vi "Scope_AM_PID_tester.vi"() -> ()   [LabVIEW 2013]
uses:
  <vilib>/rvi/interface/nirviCloseFPGA/nirviCloseFPGA.xnode
  <vilib>/rvi/interface/nirviOpenFPGA/nirviOpenFPGA.xnode
  Scope5782/Config/FPGAref_5782.ctl
  Scope/controls/Data_calc_mode.ctl
  Utilities/Ticker/Ticker.lvclass
  Scope/controls/ScopeMode.ctl
  <vilib>/rvi/interface/nirviReadWriteControl/nirviReadWriteControl.xnode
  <vilib>/Utility/error.llb/Error Cluster From Error Code.vi
  <vilib>/rvi/interface/Simulation/niFpgaSimulationCallBeginRW.vi
  <vilib>/rvi/errors/niLvFpgaAdjustHostInterfaceError.vi
  NiFpgaLv.dll
  Communication/Driver/TcpServerDriver/TcpServerDriver.lvclass
  Communication/driver_status.ctl
  Communication/response.ctl
  Communication/global_stop.vi
  Communication/Driver/RemoteConnection/RemoteConnection.lvclass
  Communication/Driver/RemoteConnection/RemoteReferences.ctl
  FPGA/fpga_settings.ctl
  <vilib>/rvi/interface/nirviMethod/nirviMethod.xnode
  <vilib>/FPGAPlugInAG/Dynamic/niLvFpga_WriteFifo_Dynamic.vi
  <vilib>/rvi/errors/niLvFpgaMergeErrorWithErrorCode.vi
  <vilib>/rvi/FXPMathLib/FxpInterpret/XNode/nifxpmath_Interpret.xnode
  <vilib>/FPGAPlugInAG/Dynamic/niLvFpga_Close_Dynamic.vi
  FPGA/DataMode.ctl
  Scope5782/Scope/controls/5782_trigger_type.ctl
  FPGA Bitfiles/AM_PID_tester_3_LzNp9O2tiLo.lvbitx
  <vilib>/FPGAPlugInAG/PXIe-7975R/niLvFpga_Open_PXIe-7975R.vi
  <vilib>/rvi/interface/common/dynamic/niFpgaDynamicAddResources.vi
  <vilib>/userdefined/High Color/nirio_resource_hc.ctl
  <vilib>/Analysis/4window.llb/windowTd.ctl
  <vilib>/Analysis/NI_AALPro.lvlib
  Scope/controls/power_spectrum_unit.ctl
  Scope/controls/graph_controls.ctl
  Scope/controls/Graph_references.ctl
  Scope/controls/Channel_select.ctl
  Scope/controls/Data_display_mode.ctl
panel:
  in  "frequency [MHz]":dbl=0.04
  in  "Ch1 deltaF":bool
  in  "c(t)":bool
  in  "Kp":fxp<+/-,32,4>
  in  "Kd/T":fxp<+/-,32,4>
  in  "Ki*T":fxp<+/-,32,4>
  in  "Feedback":bool
  in  "#bins":i32=1 min=1 max=16
  in  "Chart length":i32=200000
  in  "Trigmode":enum32{"Triggered", "Continuous"}(radio)
  in  "Refence for phase":T1
  in  "Graph_refs":T2
  out "Lower chart":dbl[][](graph)
  out "Upper chart":dbl[][](graph)
  out "Lower graph":i16[][](graph)
  in  "Buffer":T4
  in  "Display":T5
  in  "Ch1 Q":bool
  in  "Ch1 I":bool
  in  "Ch0 Q":bool
  in  "Ch0 I":bool
  in  "Ch1":bool
  in  "Ch0":bool
  out "stop 2":bool
  in  "Zoom freq X":bool
  in  "Zoom freq Y":bool
  in  "Zoom time Y":bool
  in  "Zoom time X":bool
  in  "Unit":T6
  in  "Window":T7=1 items=["Rectangle"=0, "Hanning"=1, "Hamming"=2, "Blackman-Harris"=3, "Exact Blackman"=4, "Blackman"=5, "Flat Top"=6, "4 Term B-Harris "=7, "7 Term B-Harris"=8, "Low Sidelobe"=9, "Blackman Nuttall"=11, "Triangle"=30, "Bartlett-Hanning"=31, "Bohman"=32, "Parzen"=33, "Welch"=34, "Kaiser"=60, "Dolph-Chebyshev"=61, "Gaussian"=62]
  in  "Samples per 5782 record":i32
  out "freqdata":cluster{"f0":dbl, "df":dbl, "magnitude":dbl[]}[](graph)
  out "Upper graph":i16[][](graph)
  in  "Rumode":bool
  in  "Singleshot":bool
  out "error IO":errorcluster
  in  "stop":bool
  in  "resource name":T8="RIO0"
  out "Clocking Option Configured?":bool
  out "Configured?":bool
  # "Auto Zoom"
  # "5782"
  # "FFT"
  # "Auto Zoom"
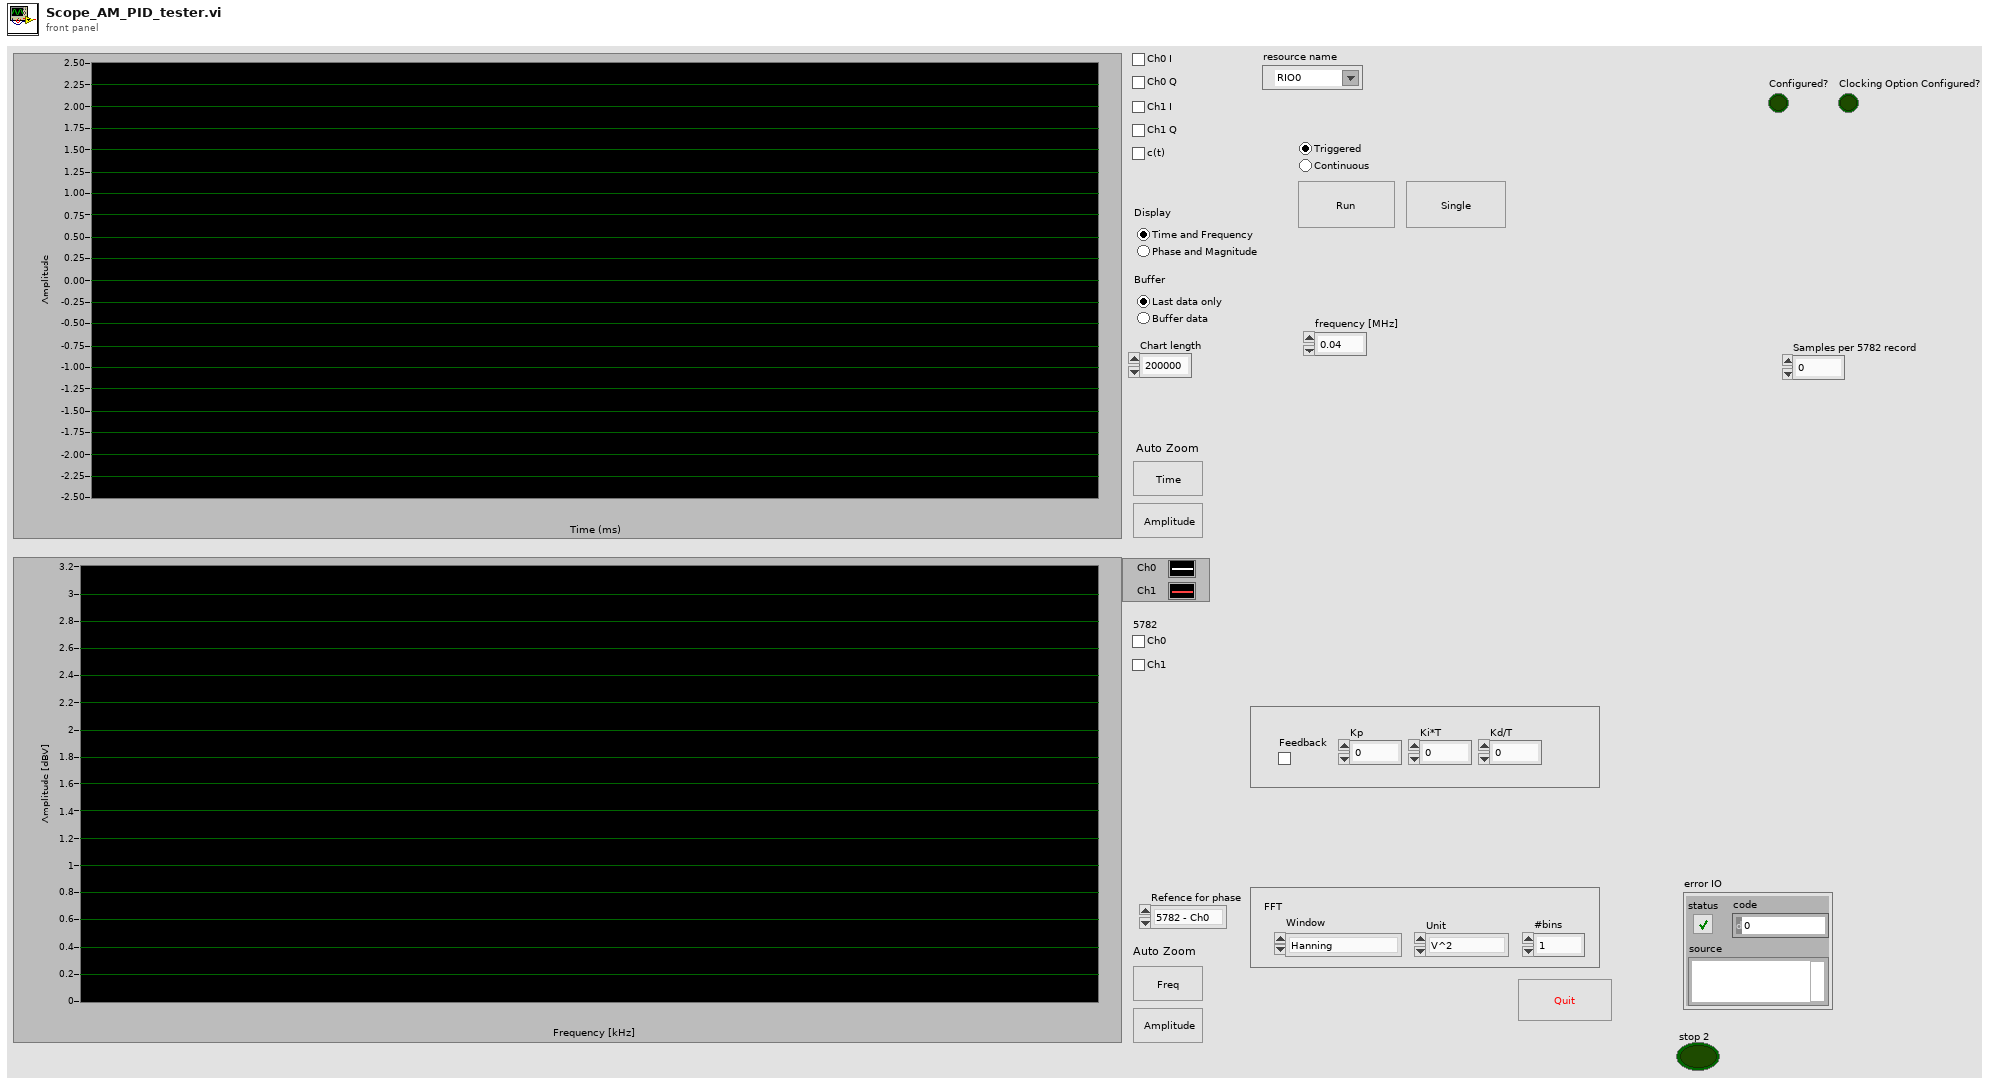
[diagram p1: front panel]
types:
  T1 = typedef "Channel_select.ctl" = enum16{"5782 - Ch0", "5782 - Ch1"}
  T2 = typedef "Graph_references.ctl" = cluster{"upper":T3, "lower":T3, "Freq graph":refnum<vi>}
  T3 = typedef "graph_controls.ctl" = cluster{"Graph":refnum<vi>, "Time btn":refnum<vi>, "Amplitude btn":refnum<vi>, "Chart":refnum<vi>}
  T4 = typedef "Data_display_mode.ctl" = enum32{"Last data only", "Buffer data"}
  T5 = typedef "Data_calc_mode.ctl" = enum32{"Time and Frequency", "Phase and Magnitude"}
  T6 = typedef "power_spectrum_unit.ctl" = enum16{"V^2", "V", "dBV"}
  T7 = typedef "NI_AALPro.lvlib/windowTd.ctl" = u32
  T8 = typedef "nirio_resource_hc.ctl" = tag
  T9 = typedef "5782_trigger_type.ctl" = enum16{"Software", "Trigger input"}
  T10 = typedef "DataMode.ctl" = enum16{"Real IO", "Simulated"}
  T11 = typedef "RemoteConnection.lvclass/RemoteReferences.ctl" = cluster{"a":refnum<vi>, "b":refnum<vi>, "fm":refnum<vi>, "Output delay":refnum<vi>, "Output delay delta":refnum<vi>}
  T12 = typedef "response.ctl" = cluster{"driver status":T13, "Sender":string, "Type":i32, "Variant":variant}
  T13 = typedef "driver_status.ctl" = enum16{"Normal", "Startup", "Connection lost", "Reconnected", "Timeout", "Idle", "Busy"}
  T14 = enum8{"Internal Clock PLL Off", "Internal Clock PLL On (REF IN)", "External Clock (CLK_IN)", "Internal Clock PLL On (IoModSyncClk)"}
  T15 = typedef "message_queue.ctl" = refnum<queue>
  T16 = typedef "FPGAref_config.ctl" = refnum<k20>
  T17 = typedef "FPGAref_5782.ctl" = refnum<k20>
  T18 = typedef "FPGAref_5782_DMA.ctl" = refnum<k20>
  T19 = typedef "scope_params_5782.ctl" = cluster{"scope mode":T20, "ticker":refnum<class "Ticker.lvclass">, "samples per record":i32, "FPGA ref":T17, "data mode":T10, "5782 Trigger":T9, "Chart length":i32, "RemoteConnection":refnum<class "RemoteConnection.lvclass">, "last phase":dbl[]}
  T20 = typedef "ScopeMode.ctl" = enum16{"Stopped", "Single", "Running", "Continuous"}
  T21 = typedef "fpga_settings.ctl" = enum16{"Feedback Enable", "New FIR coeffs", "FIR shift", "Enable filter", "Set Downsample", "Downsample", "CIC Gain", "Record length", "Trigger samples", "Quiet time", "a_am", "b_am", "Use fixed delay", "fixed sin_fi", "fixed cos_fi", "Ki*Tau", "Kp", "Kd_Tau", "Fi_start", "Fi_delta", "DC_offs 0", "DC_offs 1", "DC_offs 2", "DC_offs 3", "Ki*Tau am", "Kp am", "Kd_Tau am", "Feedback AM"}
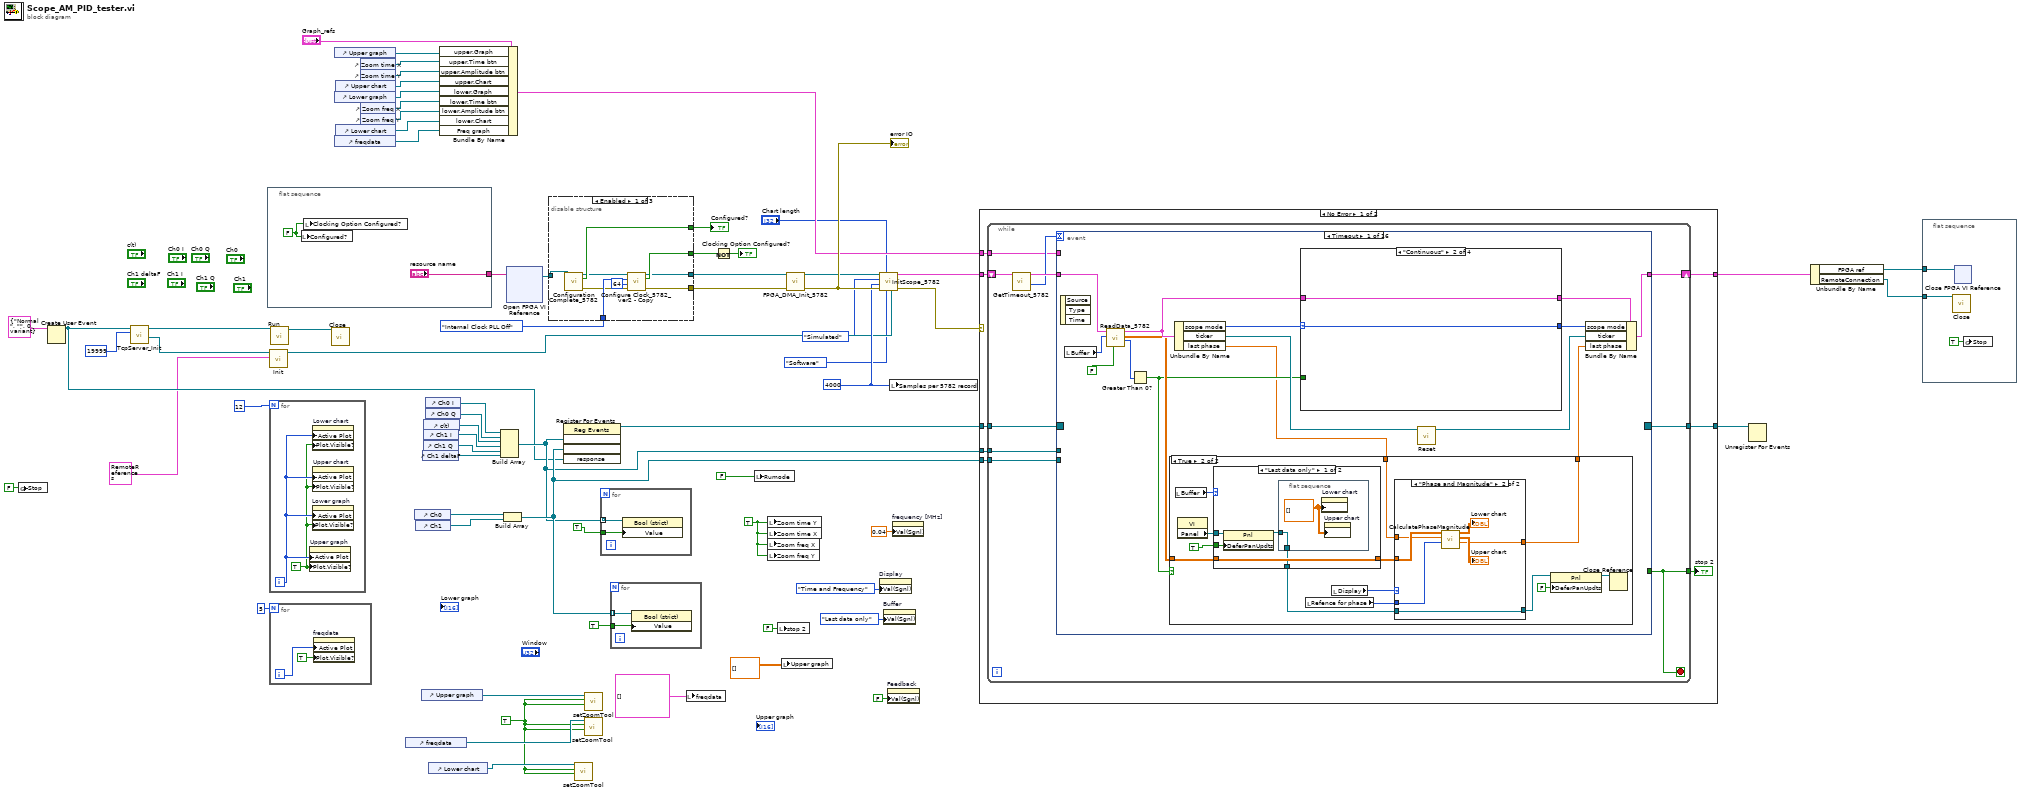
[diagram p0: block diagram]
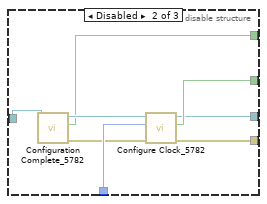
[diagram p2: hidden frame]
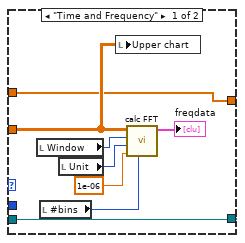
[diagram p6: hidden frame]
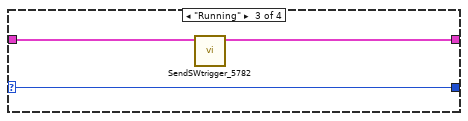
[diagram p8: hidden frame]
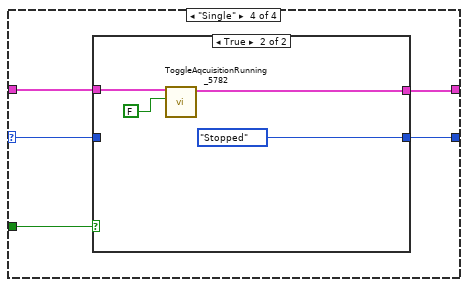
[diagram p9: hidden frame]
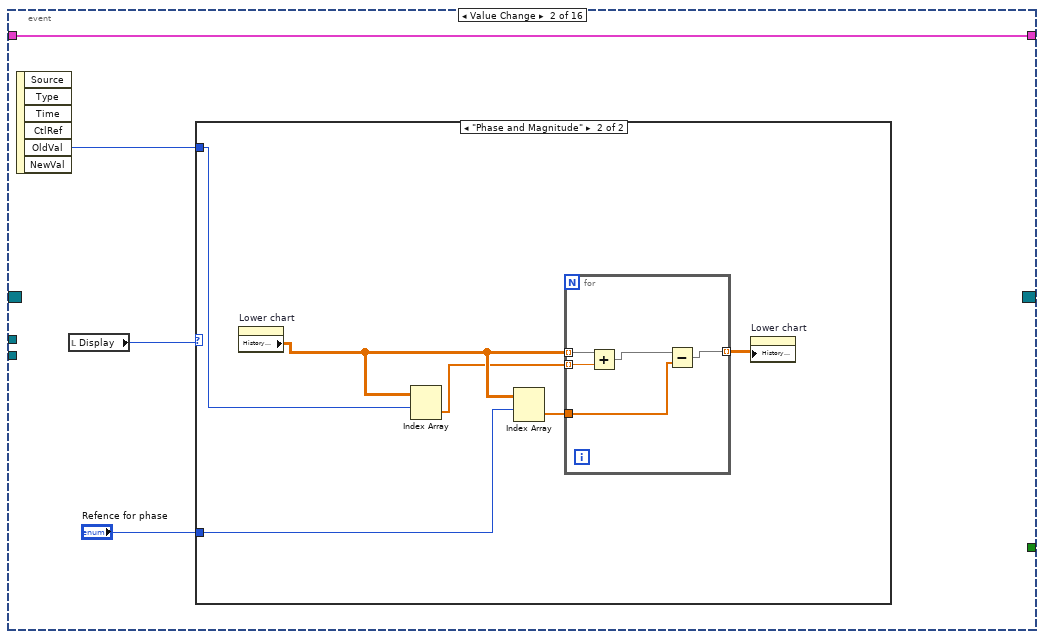
[diagram p11: hidden frame]
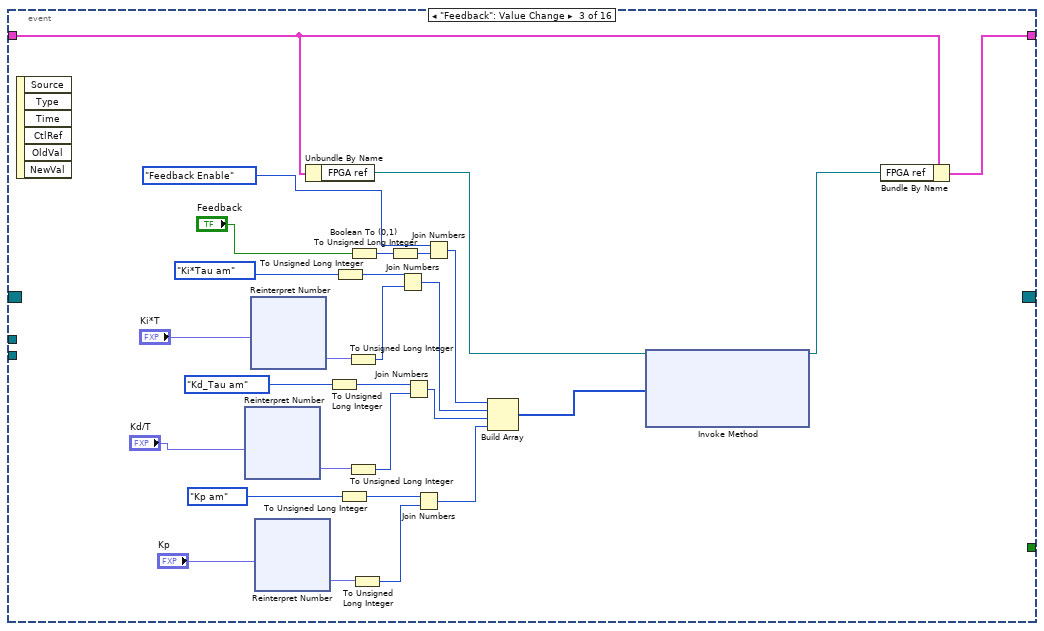
[diagram p13: hidden frame]
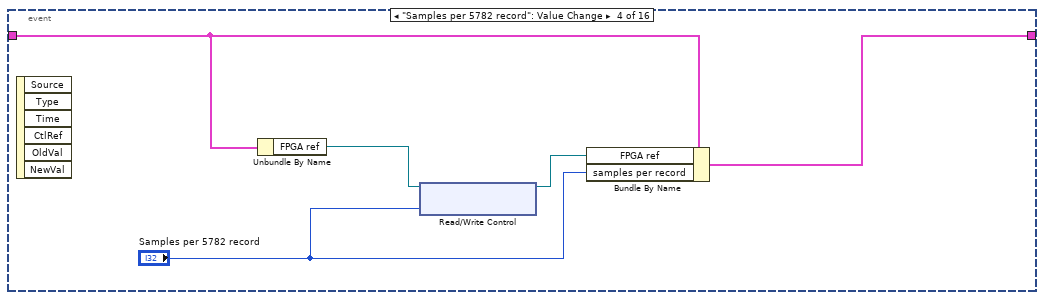
[diagram p14: hidden frame]
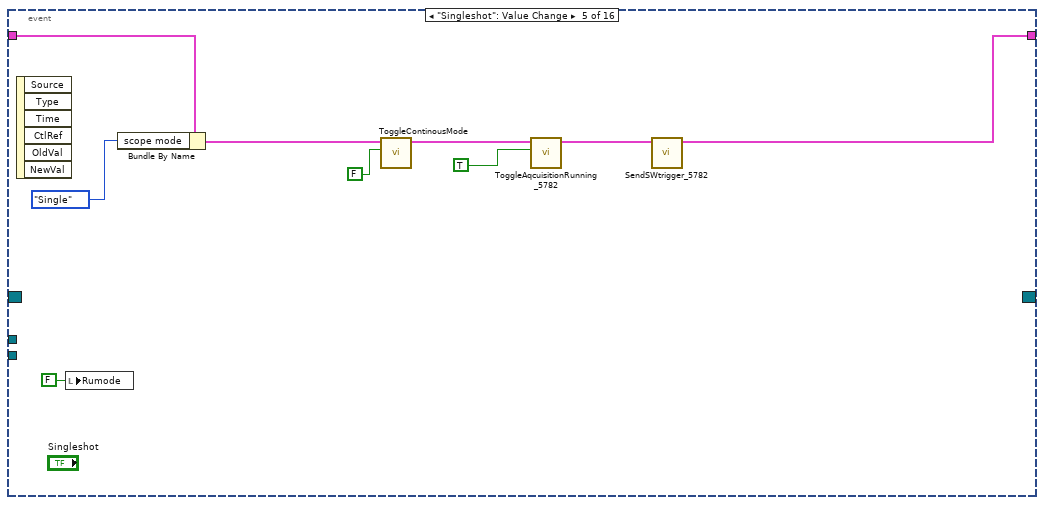
[diagram p15: hidden frame]
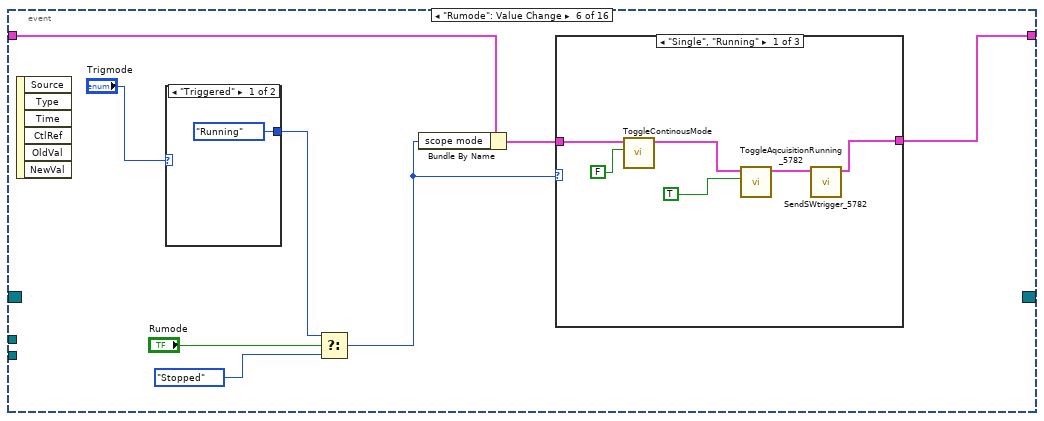
[diagram p16: hidden frame]
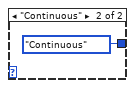
[diagram p17: hidden frame]
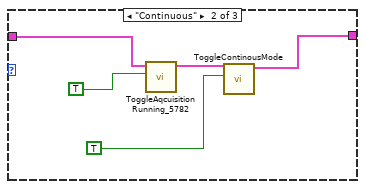
[diagram p18: hidden frame]
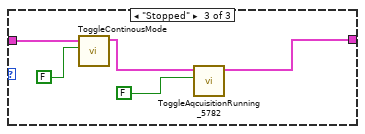
[diagram p19: hidden frame]
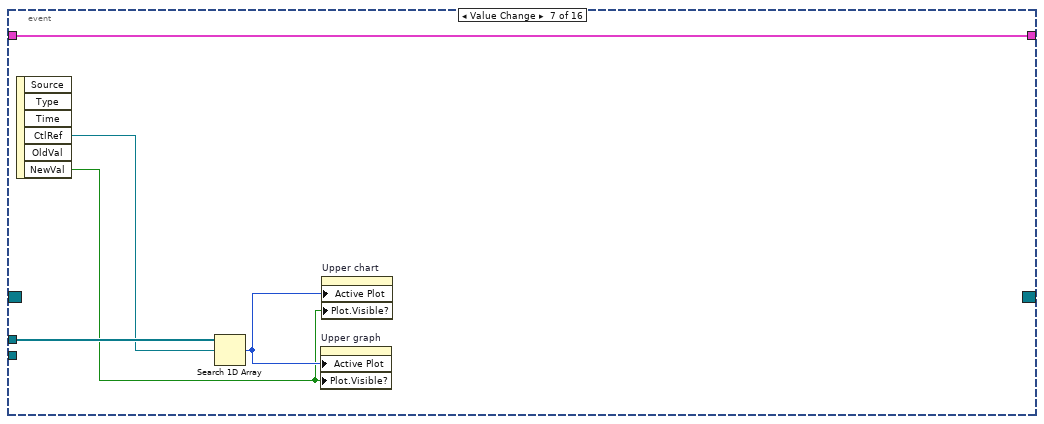
[diagram p20: hidden frame]
diagram:
  w11 = TRUE ("Zoom  X")
  w54 = TRUE ("Rumode")
  w42 = 4000 ("Samples to aqcuire")
  n1 = global write "global_stop.vi" "Stop"(FALSE ("Stop")) -> ()
  n2 = Create User Event(user event datatype=T12 {"driver status"=enum."Normal", "Sender"="", "Type"=0, "Variant"=variant} ("response")) -> (user event=w17:refnum<user-event>)  [unwired: 1 in, 1 out]
  n3 = call "TcpServer_Init.vi"("local port"=u16 19999, "response event"=w17) -> ("Message queue"=w22:T15, "TcpServerDriver"=w19:refnum<class "TcpServerDriver.lvclass">)  [unwired: 8 in]
  n4 = flat-sequence {
    tunnel: ["resource name"] -> w55
    frame #0 {
      w69 = FALSE ("Trigger Acquisition")
      n5 = local write "Configured?"(w69) -> ()
      n6 = local write "Clocking Option Configured?"(w69) -> ()
    }
  }
  n7 = call "Init.vi"("refs"=T11 {"a"=refnum, "b"=refnum, "fm"=refnum, "Output delay"=refnum, "Output delay delta"=refnum}, "server queue"=w22) -> ("RemoteConnection"=w16:refnum<class "RemoteConnection.lvclass">)  [unwired: 9 in]
  n8 = for {
    N: 12 -> [_]
    i -> [w72]
    w71 = TRUE ("Plot.Visible")
    n9 = property on="Upper graph" class="WFGraph (strict)"("Active Plot"=w72, "Plot.Visible?"=w71) -> ()  [unwired: 2 in, 2 out]
    n10 = property on="Lower graph" class="WFGraph (strict)"("Active Plot"=w72, "Plot.Visible?"=w71) -> ()  [unwired: 2 in, 2 out]
    n11 = property on="Lower chart" class="WFChart (strict)"("Active Plot"=w72, "Plot.Visible?"=w71) -> ()  [unwired: 2 in, 2 out]
    n12 = property on="Upper chart" class="WFChart (strict)"("Active Plot"=w72, "Plot.Visible?"=w71) -> ()  [unwired: 2 in, 2 out]
  }
  n13 = for {
    N: 5 -> [_]
    i -> [w73]
    n14 = property on="freqdata" class="WFGraph (strict)"("Active Plot"=w73, "Plot.Visible?"=TRUE ("Plot.Visible")) -> ()  [unwired: 2 in, 2 out]
  }
  n15 = call-dynamic "Run.vi"("BaseDriver in"=w19) -> ("BaseDriver out"=w20:refnum<class "TcpServerDriver.lvclass">)  [unwired: 9 in, 1 out]
  n16 = call-dynamic "Close.vi"("BaseDriver in"=w20) -> ()  [unwired: 9 in, 2 out]
  n17 = control-ref of="Upper graph"() -> (w39:refnum<vi>)
  n18 = control-ref of="Lower graph"() -> (w35:refnum<vi>)
  n19 = control-ref of="freqdata"() -> (w31:refnum<vi>)
  n20 = control-ref of="Upper chart"() -> (w36:refnum<vi>)
  n21 = control-ref of="Lower chart"() -> (w32:refnum<vi>)
  n22 = control-ref of="Zoom time X"() -> (w38:refnum<vi>)
  n23 = control-ref of="Zoom time Y"() -> (w37:refnum<vi>)
  n24 = control-ref of="Zoom freq X"() -> (w34:refnum<vi>)
  n25 = control-ref of="Zoom freq Y"() -> (w33:refnum<vi>)
  n26 = control-ref of="freqdata"() -> (w44:refnum<vi>)
  n27 = control-ref of="Ch0"() -> (w51:refnum<vi>)
  n28 = control-ref of="Ch1"() -> (w52:refnum<vi>)
  n29 = control-ref of="Upper graph"() -> (w45:refnum<vi>)
  n30 = control-ref of="Ch1 deltaF"() -> (w9:refnum<vi>)
  n31 = control-ref of="Ch1 I"() -> (w49:refnum<vi>)
  n32 = control-ref of="Ch1 Q"() -> (w50:refnum<vi>)
  n33 = control-ref of="c(t)"() -> (w10:refnum<vi>)
  n34 = control-ref of="Ch0 I"() -> (w47:refnum<vi>)
  n35 = control-ref of="Ch0 Q"() -> (w48:refnum<vi>)
  n36 = control-ref of="Lower chart"() -> (w12:refnum<vi>)
  n37 = Bundle By Name(cluster="Graph_refs", "upper.Graph"=w39, "upper.Time btn"=w38, "upper.Amplitude btn"=w37, "upper.Chart"=w36, "lower.Graph"=w35, "lower.Time btn"=w34, "lower.Amplitude btn"=w33, "lower.Chart"=w32, "Freq graph"=w31) -> (w30:T2)
  n38 = Build Array(w47, w48, w10, w49, w50, w9) -> (w46:refnum<vi>[])
  n39 = Build Array(w51, w52) -> (w57:refnum<vi>[])
  n40 = xnode "Open FPGA VI Reference"("resource name"=w55) -> ("FPGA VI Reference Out"=w25:refnum<k20>)  [unwired: 1 in, 1 out]
  n41 = disable-structure shown="Enabled" {
    disable-tunnel: [w83 w91 _] -> w26
    disable-tunnel: T14."Internal Clock PLL Off" ("Clock Source") -> [w82 w90 _]
    disable-tunnel: [w80 w88 _] -> w7
    disable-tunnel: [w79 w85 w92] -> w8
    disable-tunnel: w25 -> [w75 w87 w92]
    disable-tunnel: [w78 w84 _] -> w23
    frame Enabled {
      n42 = call "Configuration Complete_5782.vi"("FPGA VI Reference in"=w75) -> ("error out"=w81:errorcluster, "Configured?"=w78:bool, "FPGA VI Reference out"=w77:T16)  [unwired: 8 in]
      n43 = call "Configure Clock_5782_ver2 - Copy.vi"("error in"=w81, "User Data 1"=u8 64, "Clock Source"=w82, "FPGA VI Reference"=w77) -> ("error out"=w80:errorcluster, "Configuration Error"=w83:bool, "FPGA VI Reference out"=w79:T16)  [unwired: 5 in]
    }
    frame Disabled {
      n44 = call "Configuration Complete_5782.vi"("FPGA VI Reference in"=w87) -> ("error out"=w89:errorcluster, "Configured?"=w84:bool, "FPGA VI Reference out"=w86:T16)  [unwired: 8 in]
      n45 = call "Configure Clock_5782.vi"("error in"=w89, "Clock Source"=w90, "FPGA VI Reference in"=w86) -> ("error out"=w88:errorcluster, "Configuration Error"=w91:bool, "FPGA VI Reference Out"=w85:T17)  [unwired: 6 in]
    }
    frame Disabled {
    }
  }
  "Configured?" <- w23
  n46 = register-events(w46, w57, w17) -> (reference out=w61:refnum<event-registration>)  [unwired: 2 in, 1 out]
  n47 = call "setZoomTool.vi"("Zoom Y"=w11, "Zoom  X"=w11, "reference"=w12) -> ()  [unwired: 9 in]
  n48 = call "setZoomTool.vi"("Zoom Y"=w11, "Zoom  X"=w11, "reference"=w44) -> ()  [unwired: 9 in]
  n49 = call "setZoomTool.vi"("Zoom Y"=w11, "Zoom  X"=w11, "reference"=w45) -> ()  [unwired: 9 in]
  n50 = for {
    tunnel: w46 -> [w94] mode=indexing
    tunnel: TRUE ("Rumode") -> [w93]
    n51 = property class="Bool (strict)"(reference=w94, "Value"=w93) -> ()  [unwired: 1 in, 2 out]
  }
  n52 = for {
    tunnel: w57 -> [w96] mode=indexing
    tunnel: TRUE ("Rumode") -> [w95]
    n53 = property class="Bool (strict)"(reference=w96, "Value"=w95) -> ()  [unwired: 1 in, 2 out]
  }
  n54 = local write "freqdata"(cluster{"f0":dbl, "df":dbl, "magnitude":dbl[]}[] [] ("freqdata")) -> ()
  n55 = Not(x=w26) -> (.not. x?=→"Clocking Option Configured?":bool)
  n56 = local write "Rumode"(FALSE ("Rumode")) -> ()
  n57 = local write "Zoom time Y"(w54) -> ()
  n58 = local write "Zoom time X"(w54) -> ()
  n59 = local write "Zoom freq X"(w54) -> ()
  n60 = local write "Zoom freq Y"(w54) -> ()
  n61 = local write "stop 2"(FALSE ("stop 2")) -> ()
  n62 = local write "Upper graph"(dbl[][] [] ("Timedata")) -> ()
  n63 = call "FPGA_DMA_Init_5782.vi"("error in (no error)"=w7, "FPGA VI Reference"=w8) -> ("error out"=w43:errorcluster, "FPGA VI Out"=w4:T18)  [unwired: 7 in, 1 out]
  "error IO" <- w43
  n64 = call "InitScope_5782.vi"("RemoteConnection"=w16, "Trigger"=5782_trigger_type."Software", "Chart length"="Chart length", "error in"=w43, "Samples Per Trigger"=w42, "data mode"=DataMode."Simulated", "FPGA ref"=w4) -> ("error out"=w13:errorcluster, "scope params"=w68:T19)  [unwired: 3 in]
  n65 = property on="Display" class="RadioBtnsControl (strict)"("Val(Sgnl)"=Data_calc_mode."Time and Frequency" ("Value (Signaling)")) -> ()  [unwired: 2 in, 2 out]
  n66 = property on="Buffer" class="RadioBtnsControl (strict)"("Val(Sgnl)"=enum32{"Last data only", "Buffer data"}."Last data only" ("Value (Signaling)")) -> ()  [unwired: 2 in, 2 out]
  n67 = property on="Feedback" class="Bool (strict)"("Val(Sgnl)"=FALSE ("Value (Signaling)")) -> ()  [unwired: 2 in, 2 out]
  n68 = local write "Samples per 5782 record"(w42) -> ()
  n69 = property on="frequency [MHz]" class="DigNum (strict)"("Val(Sgnl)"=0.04 ("Value (Signaling)")) -> ()  [unwired: 2 in, 2 out]
  n70 = case shown="No Error" w13 {
    tunnel: w68 -> [w104 w333]
    tunnel: [w103 w333] -> w41
    tunnel: w61 -> [w102 w332]
    tunnel: [w101 w332] -> w60
    tunnel: w46 -> [w100 _]
    tunnel: w57 -> [w99 _]
    tunnel: w30 -> [w97 _]
    frame No Error {
      n71 = while {
        shift-right: [w114] -> w103
        shift-left: w104 -> [w113]
        tunnel: w102 -> [w110]
        tunnel: [w109] -> w101
        tunnel: w100 -> [w108]
        tunnel: w99 -> [w107]
        tunnel: [w106] -> w98
        tunnel: w97 -> [w105]
        stop <- w106 stop-if-true
        n72 = call "GetTimeout_5782.vi"("scope in"=w113) -> ("Time left"=w111:i32, "scope out"=w112:T19)  [unwired: 9 in]
        n73 = event shown="[0] Timeout" {
          selector: w110 -> [_ _ _ _ _ _ _ _ _ _ _ _ _ _ _ _]
          dyn-events: [_ _ _ _ _ _ _ _ _ _ _ _ _ _ _ _] -> w109
          timeout: w111 -> [_ _ _ _ _ _ _ _ _ _ _ _ _ _ _ _]
          tunnel: [_ _ _ _ _ _ _ _ _ "stop" _ _ _ _ _ _] -> w106
          tunnel: w112 -> [w124 w189 w228 w230 w240 w248 w273 w278 w283 w286 w293 w303 w308 w314 w321 w324]
          tunnel: [w127 w189 w227 w229 w237 w245 w273 w278 w282 w286 w293 w303 w308 w314 w321 w322] -> w114
          tunnel: w108 -> [_ _ _ _ _ _ w272 _ _ _ _ _ _ _ _ _]
          tunnel: w107 -> [_ _ _ _ _ _ _ w276 _ _ _ _ _ _ _ _]
          tunnel: w105 -> [_ _ _ _ _ _ _ _ _ _ _ _ _ _ w318 _]
          event Timeout {
            n74 = event-data() -> ()  [unwired: 1 in, 3 out]
            n75 = local read "Buffer"() -> (w118:T4)
            n76 = call "ReadData_5782.vi"("c(t)"=FALSE ("c(t) phase"), "Buffer mode"=w118, "scope params"=w124) -> ("Num elements"=w120:i32, "data"=w121:dbl[][], "scope params out"=w123:T19)  [unwired: 6 in]
            n77 = Greater Than 0?(x=w120) -> (x > 0?=w119:bool)
            n78 = Unbundle By Name(w123) -> ("scope mode"=w126:T20, "ticker"=w129:refnum<class "Ticker.lvclass">, "last phase"=w117:dbl[])
            n79 = case shown="True" w119 {
              tunnel: w121 -> [_ w140]
              tunnel: w117 -> [w130 w132]
              tunnel: [w130 w131] -> w116
              frame False {
              }
              frame True {
                n80 = local read "Buffer"() -> (w142:T4)
                n81 = property class="VI"() -> ("Panel"=w135:refnum<vi>)  [unwired: 2 in, 2 out]
                n82 = case shown="\"Last data only\"" w142 {
                  tunnel: w140 -> [w148 w152]
                  tunnel: [w148 w152] -> w141
                  tunnel: w135 -> [w147 w151]
                  tunnel: TRUE ("Defer Panel Updates") -> [w145 _]
                  tunnel: [w144 w151] -> w133
                  frame "Last data only" {
                    n83 = property class="Pnl"(reference=w147, "DeferPanUpdts"=w145) -> (reference out=w146:refnum<vi>)  [unwired: 1 in, 1 out]
                    n84 = flat-sequence {
                      tunnel: w146 -> [w149]
                      tunnel: [w149] -> w144
                      frame #0 {
                        w150 = dbl[][] [] ("History Data")
                        n85 = property on="Lower chart" class="WFChart (strict)"("History Data"=w150) -> ()  [unwired: 2 in, 2 out]
                        n86 = property on="Upper chart" class="WFChart (strict)"("History Data"=w150) -> ()  [unwired: 2 in, 2 out]
                      }
                    }
                  }
                  frame "Buffer data" {
                  }
                }
                n87 = local read "Refence for phase"() -> (w139:T1)
                n88 = local read "Display"() -> (w143:T5)
                n89 = case shown="\"Phase and Magnitude\"" w143 {
                  tunnel: w141 -> [w156 w167]
                  tunnel: w139 -> [_ w164]
                  tunnel: [w155 w163] -> w137
                  tunnel: w133 -> [w155 w163]
                  tunnel: w132 -> [w153 w162]
                  tunnel: [w153 w161] -> w131
                  frame "Time and Frequency" {
                    n90 = local read "Window"() -> (w157:T7)
                    n91 = local read "#bins"() -> (w154:i32)
                    n92 = local read "Unit"() -> (w158:T6)
                    n93 = local write "Upper chart"(w156) -> ()
                    n94 = call "calc FFT.vi"("#bins"=w154, "dt"=1e-06, "Unit"=w158, "Window"=w157, "data"=w156) -> ("Power Spectrum / PSD"=→"freqdata":cluster{"f0":dbl, "df":dbl, "magnitude":dbl[]}[])  [unwired: 6 in]
                  }
                  frame "Phase and Magnitude" {
                    n95 = call "CalculatePhaseMagnitude.vi"("phase reference channel"=w164, "previous phase"=w162, "data"=w167) -> ("last phase"=w161:dbl[], "Magnitude"=→"Upper chart":dbl[][], "Phase"=→"Lower chart":dbl[][])  [unwired: 6 in]
                  }
                }
                n96 = property class="Pnl"(reference=w137, "DeferPanUpdts"=FALSE ("Defer Panel Updates")) -> (reference out=w136:refnum<vi>)  [unwired: 1 in, 1 out]
                n97 = Close Reference(reference=w136) -> ()  [unwired: 1 in, 1 out]
              }
            }
            n98 = case shown="\"Continuous\"" w126 {
              selector: w126 -> [w169 w171 w174 w175]
              tunnel: [w169 w171 w174 w179] -> w125
              tunnel: w123 -> [w168 w170 w173 w177]
              tunnel: [w168 w170 w172 w176] -> w122
              tunnel: w119 -> [_ _ _ w178]
              frame "Stopped" {
              }
              frame "Continuous" {
              }
              frame "Running" {
                n99 = call "SendSWtrigger_5782.vi"("scope in"=w173) -> ("scope out"=w172:T19)  [unwired: 9 in, 1 out]
              }
              frame "Single" {
                n100 = case shown="True" w178 {
                  tunnel: [w180 ScopeMode."Stopped" ("scope mode")] -> w179
                  tunnel: w177 -> [w181 w184]
                  tunnel: [w181 w183] -> w176
                  tunnel: w175 -> [w180 _]
                  frame False {
                  }
                  frame True {
                    n101 = call "ToggleAqcuisitionRunning_5782.vi"("Acquisition running"=FALSE, "scope in"=w184) -> ("scope out"=w183:T19)  [unwired: 8 in, 1 out]
                  }
                }
              }
            }
            n102 = call "Reset.vi"("Ticker in"=w129) -> ("Ticker out"=w128:refnum<class "Ticker.lvclass">)  [unwired: 9 in, 1 out]
            n103 = Bundle By Name(cluster=w122, "scope mode"=w125, "ticker"=w128, "last phase"=w116) -> (w127:T19)
          }
          event Value Change {
            n104 = event-data() -> ("OldVal"=w186:T1)  [unwired: 1 in, 5 out]
            n105 = local read "Display"() -> (w187:T5)
            n106 = case shown="\"Phase and Magnitude\"" w187 {
              tunnel: "Refence for phase" -> [_ w194]
              tunnel: w186 -> [_ w192]
              frame "Time and Frequency", Default {
              }
              frame "Phase and Magnitude" {
                n107 = property on="Lower chart" class="WFChart (strict)"() -> ("History Data"=w193:dbl[][])  [unwired: 2 in, 2 out]
                n108 = Index Array(array=w193, index (row)=w192) -> (element=w191:dbl[])  [unwired: 1 in]
                n109 = Index Array(array=w193, index (row)=w194) -> (element=w195:dbl[])  [unwired: 1 in]
                n110 = for {
                  tunnel: w193 -> [w198] mode=indexing
                  tunnel: w195 -> [w200]
                  tunnel: [w199] -> w190 mode=indexing
                  tunnel: w191 -> [w197] mode=indexing
                  n111 = Add(x=w198, y=w197) -> (x+y=w196:dbl[])
                  n112 = Subtract(x=w196, y=w200) -> (x-y=w199:dbl[])
                }
                n113 = property on="Lower chart" class="WFChart (strict)"("History Data"=w190) -> ()  [unwired: 2 in, 2 out]
              }
            }
          }
          event "Feedback": Value Change {
            n114 = event-data() -> ()  [unwired: 1 in, 6 out]
            n115 = xnode "Reinterpret Number"("x"="Kd/T") -> ("y"=w214:fxp<+,32,32>)
            n116 = xnode "Reinterpret Number"("x"="Ki*T") -> ("y"=w211:fxp<+,32,32>)
            n117 = xnode "Reinterpret Number"("x"="Kp") -> ("y"=w218:fxp<+,32,32>)
            n118 = Unbundle By Name(w228) -> ("FPGA ref"=w226:T17)
            n119 = To Unsigned Long Integer(number=fpga_settings."Kd_Tau am" ("FPGA Setting")) -> (unsigned 32bit integer=w212:u32)
            n120 = To Unsigned Long Integer(number=fpga_settings."Ki*Tau am" ("FPGA Setting")) -> (unsigned 32bit integer=w208:u32)
            n121 = To Unsigned Long Integer(number=fpga_settings."Kp am" ("FPGA Setting")) -> (unsigned 32bit integer=w215:u32)
            n122 = To Unsigned Long Integer(number=w211) -> (unsigned 32bit integer=w207:u32)
            n123 = To Unsigned Long Integer(number=w214) -> (unsigned 32bit integer=w213:u32)
            n124 = Boolean To (0,1)(Boolean="Feedback") -> (0, 1=w223:i16)
            n125 = To Unsigned Long Integer(number=w218) -> (unsigned 32bit integer=w217:u32)
            n126 = To Unsigned Long Integer(number=w223) -> (unsigned 32bit integer=w220:u32)
            n127 = Join Numbers(hi=w208, lo=w207) -> ((hi.lo)=w206:u64)
            n128 = Join Numbers(hi=w212, lo=w213) -> ((hi.lo)=w205:u64)
            n129 = Join Numbers(hi=w215, lo=w217) -> ((hi.lo)=w225:u64)
            n130 = Join Numbers(hi=fpga_settings."Feedback Enable" ("FPGA Setting"), lo=w220) -> ((hi.lo)=w221:u64)
            n131 = Build Array(w221, w206, w205, w225) -> (w224:u64[])
            n132 = xnode "Invoke Method"("FPGA VI Reference In"=w226, "Data"=w224) -> ("FPGA VI Reference Out"=w201:T17)  [unwired: 2 in, 2 out]
            n133 = Bundle By Name(cluster=w228, "FPGA ref"=w201) -> (w227:T19)
          }
          event "Samples per 5782 record": Value Change {
            n134 = event-data() -> ()  [unwired: 1 in, 6 out]
            n135 = Unbundle By Name(w230) -> ("FPGA ref"=w233:T17)
            n136 = xnode "Read/Write Control"("FPGA VI Reference In"=w233, "5782 record length"="Samples per 5782 record") -> ("FPGA VI Reference Out"=w232:T17)  [unwired: 1 in, 1 out]
            n137 = Bundle By Name(cluster=w230, "FPGA ref"=w232, "samples per record"="Samples per 5782 record") -> (w229:T19)
          }
          event "Singleshot": Value Change {
            n138 = event-data() -> ()  [unwired: 1 in, 6 out]
            n139 = local write "Rumode"(FALSE ("Rumode")) -> ()
            n140 = Bundle By Name(cluster=w240, "scope mode"=ScopeMode."Single") -> (w235:T19)
            n141 = call "ToggleContinousMode.vi"("Cont Acquisition"=FALSE, "scope in"=w235) -> ("scope out"=w234:T19)  [unwired: 8 in, 1 out]
            n142 = call "ToggleAqcuisitionRunning_5782.vi"("Acquisition running"=TRUE, "scope in"=w234) -> ("scope out"=w238:T19)  [unwired: 8 in, 1 out]
            n143 = call "SendSWtrigger_5782.vi"("scope in"=w238) -> ("scope out"=w237:T19)  [unwired: 9 in, 1 out]
          }
          event "Rumode": Value Change {
            n144 = event-data() -> ()  [unwired: 1 in, 6 out]
            n145 = case shown="\"Triggered\"" "Trigmode" {
              tunnel: [ScopeMode."Running" ("scope mode") ScopeMode."Continuous" ("scope mode")] -> w243
              frame "Triggered" {
              }
              frame "Continuous" {
              }
            }
            n146 = Select(t=w243, s="Rumode", f=ScopeMode."Stopped" ("scope mode")) -> (s? t:f=w247:T20)
            n147 = Bundle By Name(cluster=w248, "scope mode"=w247) -> (w246:T19)
            n148 = case shown="\"Single\", \"Running\"" w247 {
              tunnel: w246 -> [w255 w262 w266]
              tunnel: [w256 w260 w267] -> w245
              frame "Single", "Running" {
                n149 = call "ToggleContinousMode.vi"("Cont Acquisition"=FALSE, "scope in"=w255) -> ("scope out"=w253:T19)  [unwired: 8 in, 1 out]
                n150 = call "ToggleAqcuisitionRunning_5782.vi"("Acquisition running"=TRUE, "scope in"=w253) -> ("scope out"=w257:T19)  [unwired: 8 in, 1 out]
                n151 = call "SendSWtrigger_5782.vi"("scope in"=w257) -> ("scope out"=w256:T19)  [unwired: 9 in, 1 out]
              }
              frame "Continuous" {
                n152 = call "ToggleAqcuisitionRunning_5782.vi"("Acquisition running"=TRUE, "scope in"=w262) -> ("scope out"=w261:T19)  [unwired: 8 in, 1 out]
                n153 = call "ToggleContinousMode.vi"("Cont Acquisition"=TRUE ("Acquisition running"), "scope in"=w261) -> ("scope out"=w260:T19)  [unwired: 8 in, 1 out]
              }
              frame "Stopped" {
                n154 = call "ToggleContinousMode.vi"("Cont Acquisition"=FALSE, "scope in"=w266) -> ("scope out"=w264:T19)  [unwired: 8 in, 1 out]
                n155 = call "ToggleAqcuisitionRunning_5782.vi"("Acquisition running"=FALSE, "scope in"=w264) -> ("scope out"=w267:T19)  [unwired: 8 in, 1 out]
              }
            }
          }
          event Value Change {
            n156 = event-data() -> ("CtlRef"=w271:refnum<vi>, "NewVal"=w269:bool)  [unwired: 1 in, 4 out]
            n157 = Search 1D Array(1D array=w272, element=w271) -> (index of element=w270:i32)  [unwired: 1 in]
            n158 = property on="Upper graph" class="WFGraph (strict)"("Active Plot"=w270, "Plot.Visible?"=w269) -> ()  [unwired: 2 in, 2 out]
            n159 = property on="Upper chart" class="WFChart (strict)"("Active Plot"=w270, "Plot.Visible?"=w269) -> ()  [unwired: 2 in, 2 out]
          }
          event Value Change {
            n160 = event-data() -> ("CtlRef"=w277:refnum<vi>, "NewVal"=w274:bool)  [unwired: 1 in, 4 out]
            n161 = Search 1D Array(1D array=w276, element=w277) -> (index of element=w275:i32)  [unwired: 1 in]
            n162 = property on="freqdata" class="WFGraph (strict)"("Active Plot"=w275, "Plot.Visible?"=w274) -> ()  [unwired: 2 in, 2 out]
            n163 = property on="Lower chart" class="WFChart (strict)"("Active Plot"=w275, "Plot.Visible?"=w274) -> ()  [unwired: 2 in, 2 out]
          }
          event User Event {
            n164 = event-data() -> ("Sender"=w281:string, "Variant"=w280:variant, "driver status"=w279:T13)  [unwired: 1 in, 5 out]
            n165 = Unbundle By Name(w283) -> ("RemoteConnection"=w285:refnum<class "RemoteConnection.lvclass">)
            n166 = call "HandleRemoteMessage.vi"("driver status"=w279, "Message data"=w280, "Sender"=w281, "RemoteConnection in"=w285) -> ("RemoteConnection out"=w284:refnum<class "RemoteConnection.lvclass">)  [unwired: 6 in, 1 out]
            n167 = Bundle By Name(cluster=w283, "RemoteConnection"=w284) -> (w282:T19)
          }
          event "stop": Value Change {
            n168 = event-data() -> ()  [unwired: 1 in, 6 out]
          }
          event Value Change {
            n169 = event-data() -> ()  [unwired: 1 in, 6 out]
            n170 = case shown="\"V\"" "Unit" {
              tunnel: ["V" "dBV" "V^2"] -> w290
              frame "V" {
              }
              frame "dBV" {
              }
              frame "V^2" {
              }
            }
            n171 = Concatenate Strings("Amplitude [", w290, "]") -> (w288:string)
            n172 = property on="freqdata" class="WFGraph (strict)"("YScale.NameLbl.Text"=w288) -> ()  [unwired: 2 in, 2 out]
          }
          event "#bins": Value Change {
            n173 = event-data() -> ()  [unwired: 1 in, 6 out]
            n174 = local read "Upper chart"() -> (w299:dbl[][])
            n175 = local read "Window"() -> (w300:T7)
            n176 = local read "Unit"() -> (w301:T6)
            n177 = call "calc FFT.vi"("#bins"="#bins", "dt"=1e-06, "Unit"=w301, "Window"=w300, "data"=w299) -> ("Power Spectrum / PSD"=w298:cluster{"f0":dbl, "df":dbl, "magnitude":dbl[]}[])  [unwired: 6 in]
            n178 = local write "freqdata"(w298) -> ()
          }
          event "Zoom time X", "Zoom time Y": Value Change {
            n179 = event-data() -> ()  [unwired: 1 in, 6 out]
            n180 = control-ref of="Upper chart"() -> (w306:refnum<vi>)
            n181 = control-ref of="Upper graph"() -> (w307:refnum<vi>)
            n182 = call "setZoomTool.vi"("Zoom Y"="Zoom time Y", "Zoom  X"="Zoom time X", "reference"=w306) -> ()  [unwired: 9 in]
            n183 = call "setZoomTool.vi"("Zoom Y"="Zoom time Y", "Zoom  X"="Zoom time X", "reference"=w307) -> ()  [unwired: 9 in]
          }
          event "Zoom freq Y", "Zoom freq X": Value Change {
            n184 = event-data() -> ()  [unwired: 1 in, 6 out]
            n185 = control-ref of="Lower chart"() -> (w312:refnum<vi>)
            n186 = control-ref of="Lower graph"() -> (w311:refnum<vi>)
            n187 = control-ref of="freqdata"() -> (w313:refnum<vi>)
            n188 = call "setZoomTool.vi"("Zoom Y"="Zoom freq Y", "Zoom  X"="Zoom freq X", "reference"=w313) -> ()  [unwired: 9 in]
            n189 = call "setZoomTool.vi"("Zoom Y"="Zoom freq Y", "Zoom  X"="Zoom freq X", "reference"=w312) -> ()  [unwired: 9 in]
            n190 = call "setZoomTool.vi"("Zoom Y"="Zoom freq Y", "Zoom  X"="Zoom freq X", "reference"=w311) -> ()  [unwired: 9 in]
          }
          event Value Change {
            w317 = dbl[][] [] ("History Data")
            n191 = event-data() -> ()  [unwired: 1 in, 6 out]
            n192 = property on="Upper chart" class="WFChart (strict)"("History Data"=w317) -> ()  [unwired: 2 in, 2 out]
            n193 = property on="Lower chart" class="WFChart (strict)"("History Data"=w317) -> ()  [unwired: 2 in, 2 out]
            n194 = local write "freqdata"(cluster{"f0":dbl, "df":dbl, "magnitude":dbl[]}[] [] ("freqdata")) -> ()
            n195 = call "UpdateGraphs.vi"("Buffer mode"="Buffer", "Display mode"="Display", "Graph_refs"=w318) -> ()  [unwired: 9 in]
            n196 = property on="Zoom time X" class="Bool (strict)"("Val(Sgnl)"=TRUE ("Value (Signaling)")) -> ()  [unwired: 2 in, 2 out]
          }
          event "frequency [MHz]": Value Change {
            n197 = event-data() -> ()  [unwired: 1 in, 6 out]
            n198 = Unbundle By Name(w324) -> ("FPGA ref"=w326:T17)
            n199 = call "Calc phase increase and offset.vi"("# of DDS"=1, "fclk (MHz)"=10.0, "f_generated (MHz)"="frequency [MHz]") -> ("Phase out"=w329:fxp<+,64,64>[])  [unwired: 6 in, 2 out]
            n200 = Index Array(array=w329) -> (element=w327:fxp<+,64,64>)  [unwired: 1 in]
            n201 = Build Array(w327, w327) -> (w325:fxp<+,64,64>[])
            n202 = xnode "Read/Write Control"("FPGA VI Reference In"=w326, "Phase 5782"=w325) -> ("FPGA VI Reference Out"=w323:T17)  [unwired: 1 in, 1 out]
            n203 = Bundle By Name(cluster=w324, "FPGA ref"=w323) -> (w322:T19)
          }
        }
      }
      "stop 2" <- w98
    }
    frame Error {
    }
  }
  n204 = Unregister For Events(event registration refnum=w60) -> ()  [unwired: 1 in, 1 out]
  n205 = Unbundle By Name(w41) -> ("FPGA ref"=w67:T17, "RemoteConnection"=w15:refnum<class "RemoteConnection.lvclass">)
  n206 = flat-sequence {
    tunnel: w67 -> [w336]
    tunnel: w15 -> [w335]
    frame #0 {
      n207 = call "Close.vi"("RemoteConnection in"=w335) -> ()  [unwired: 9 in, 2 out]
      n208 = xnode "Close FPGA VI Reference"("FPGA VI Reference In"=w336) -> ()  [unwired: 1 in, 1 out]
      n209 = global write "global_stop.vi" "Stop"(TRUE ("Stop")) -> ()
    }
  }
